vi "Convert Error.vi"(7 "Errors":T1, 8 "error in (no error)":errorcluster, 10 "error message (\"\")":string, 11 "Error Occured?":errorcluster) -> (0 "error out":errorcluster)   [LabVIEW 2018, in "Scripting.lvlib"]
uses:
  Scripting.lvlib
  Error-Codes.ctl
  <vilib>/Utility/error.llb/Error Cluster From Error Code.vi
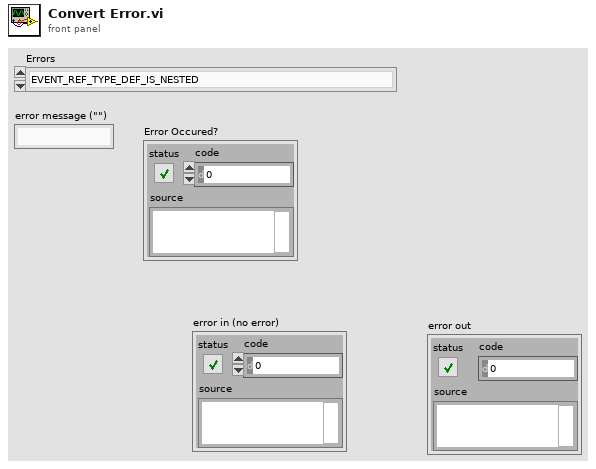
[diagram p1: front panel]
types:
  T1 = typedef "Scripting.lvlib/Error-Codes.ctl" = enum16{"EVENT_REF_TYPE_DEF_IS_NESTED", "EVENT_REF_TYPE_DEF_IS_EMPTY", "EVENT_REF_TYPE_DEF_INCLUDES_NON_REFS", "EVENT_REF_TYPE_INVALID_REPLY_REF", "EVENT_REF_TYPE_REPLY_IS_NOT_TYPE_DEF", "EVENT_REF_TYPE_DEF_IS_NOT_CLUSTER", "EVENT_REF_TYPE_DEF_INVALID_REQ_REPLY_TYPE"}
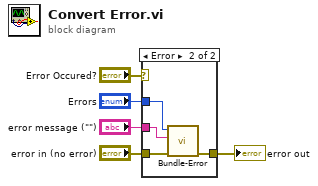
[diagram p0: block diagram]
diagram:
  n1 = case shown="Error" "Error Occured?" {
    tunnel: [w6 w9] -> w2
    tunnel: "error in (no error)" -> [w6 w10]
    tunnel: "Errors" -> [_ w8]
    tunnel: "error message (\"\")" -> [_ w7]
    frame No Error {
    }
    frame Error {
      n2 = call "Bundle-Error.vi"("error in (no error)"=w10, "error message (\"\")"=w7, "Errors"=w8) -> ("error out"=w9:errorcluster)  [unwired: 8 in]
    }
  }
  "error out" <- w2
